vi "Get Pressure Servo Valve Value.vi"(8 "error in (no error)":errorcluster, 11 "ILC Closed Loop Actuator Cylinder in":refnum<class "ILC Closed Loop Actuator Cylinder.lvclass">) -> (0 "error out":errorcluster, 2 "Value":dbl format="%.2f", 3 "ILC Closed Loop Actuator Cylinder out":refnum<class "ILC Closed Loop Actuator Cylinder.lvclass">)   [LabVIEW 2015, in "ILC Closed Loop Actuator Cylinder.lvclass"]
uses:
  ILC Closed Loop Actuator Cylinder.lvclass
  ILC Actuator Cylinder/ILC Actuator Cylinder.lvclass/ILC Actuator Cylinder.ctl
  ILC Closed Loop Actuator Cylinder.lvclass/ILC Closed Loop Actuator Cylinder.ctl
  <vilib>/addons/control/pid/pid.llb/PID (DBL).vi
  <vilib>/addons/control/pid/NI_PID_pid.lvlib
  ILC Actuator Cylinder/ILC Actuator Cylinder.lvclass
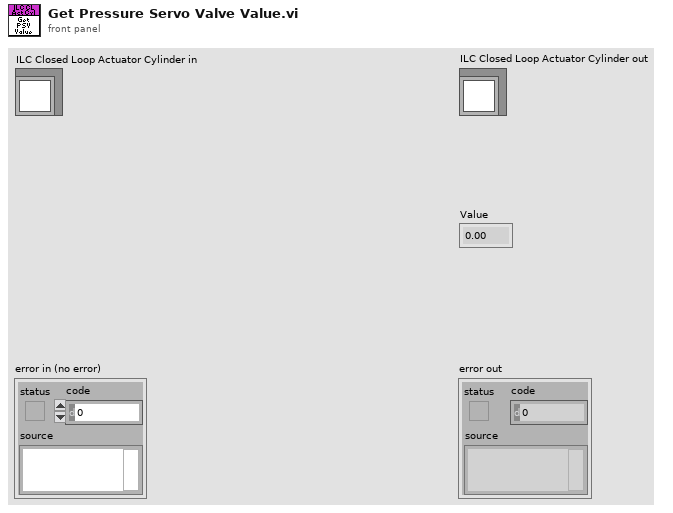
[diagram p1: front panel]
types:
  T1 = cluster{"proportional gain (Kc)":dbl, "integral time (Ti, min)":dbl, "derivative time (Td, min)":dbl}
  T2 = typedef "FAMT Typedefs.lvlib/PID Settings.ctl" = cluster{"Pressure Servo Valve Settings":T3, "Turbo Valve Settings":T3}
  T3 = typedef "FAMT Typedefs.lvlib/Closed Loop Settings.ctl" = cluster{"P":dbl, "I":dbl, "D":dbl, "Minimum":dbl, "Maximum":dbl}
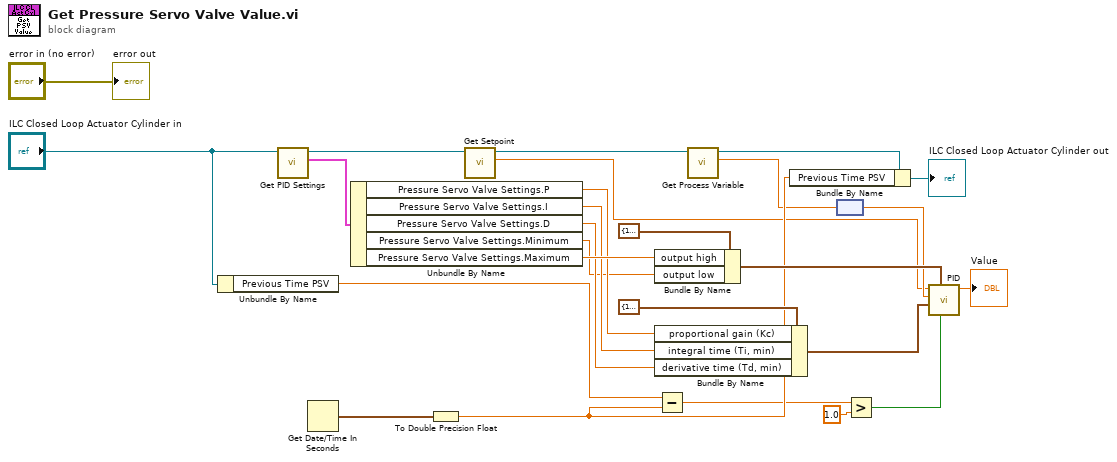
[diagram p0: block diagram]
diagram:
  n1 = Unbundle By Name("ILC Closed Loop Actuator Cylinder in") -> ("Previous Time PSV"=w7:dbl)
  n2 = call "Get PID Settings.vi"("ILC Actuator Cylinder in"="ILC Closed Loop Actuator Cylinder in") -> ("PID Settings"=w8:T2, "ILC Actuator Cylinder out"=w6:refnum<class "ILC Closed Loop Actuator Cylinder.lvclass">)  [unwired: 9 in]
  n3 = Get Date/Time In Seconds() -> (seconds since 1Jan1904=w15:timestamp)
  n4 = Unbundle By Name(w8) -> ("Pressure Servo Valve Settings.P"=w21:dbl, "Pressure Servo Valve Settings.I"=w20:dbl, "Pressure Servo Valve Settings.D"=w19:dbl, "Pressure Servo Valve Settings.Minimum"=w16:dbl, "Pressure Servo Valve Settings.Maximum"=w24:dbl)
  n5 = To Double Precision Float(number=w15) -> (double precision float=w13:dbl)
  n6 = call-dynamic "Get Setpoint.vi"("ILC Actuator Cylinder in"=w6) -> ("Setpoint"=w5:dbl, "ILC Actuator Cylinder out"=w4:refnum<class "ILC Closed Loop Actuator Cylinder.lvclass">)  [unwired: 9 in]
  n7 = Bundle By Name(cluster=cluster{"output high":dbl, "output low":dbl} {"output high"=100.0, "output low"=-100.0} ("output range"), "output high"=w24, "output low"=w16) -> (w23:cluster{"output high":dbl, "output low":dbl})
  n8 = Bundle By Name(cluster=T1 {"proportional gain (Kc)"=1.0, "integral time (Ti, min)"=0.01, "derivative time (Td, min)"=0.0} ("PID gains"), "proportional gain (Kc)"=w21, "integral time (Ti, min)"=w20, "derivative time (Td, min)"=w19) -> (w18:T1)
  n9 = Subtract(x=w7, y=w13) -> (x-y=w12:dbl)
  n10 = call-dynamic "Get Process Variable.vi"("ILC Actuator Cylinder in"=w4) -> ("Process Variable"=w1:dbl[unit], "ILC Actuator Cylinder out"=w2:refnum<class "ILC Closed Loop Actuator Cylinder.lvclass">)  [unwired: 9 in]
  n11 = Bundle By Name(cluster=w2, "Previous Time PSV"=w13) -> (→"ILC Closed Loop Actuator Cylinder out":refnum<class "ILC Closed Loop Actuator Cylinder.lvclass">)
  n12 = node(w1) -> (w17:dbl)
  n13 = Greater?(x=w12, y=1.0) -> (0:w10:bool)
  n14 = call-poly <vilib>:"PID.vi"("reinitialize? (F)"=w10, "output range"=w23, "PID gains"=w18, "process variable"=w17, "setpoint"=w5) -> ("output"=→"Value":dbl)  [unwired: 5 in, 1 out]
  "error out" <- "error in (no error)"
